vi "Inspect BBM Fiducials.vi"(5 "Dispose Images?":bool, 6 "BBM Chuck":i32, 7 "Glue Pathways":T7 {"BBM Slot" items=["Slot 1", "Slot 2", "Slot 3", "Slot 4"]; "Weight Slot" items=["Slot 1", "Slot 2", "Slot 3", "Slot 4"]; "Glue Slot" items=["Slot 1", "Slot 2", "Slot 3", "Slot 4"]; "Stamp Slot" items=["Slot 1", "Slot 2", "Slot 3", "Slot 4"]; "HDI Slot" items=["Slot 1", "Slot 2", "Slot 3", "Slot 4"]}, 8 "error in":errorcluster, 9 "Console Log in":refnum<class "Console Log.lvclass">, 10 "Single Path in":T6, 11 "CameraTool in":refnum<class "CameraTool Class.lvclass">) -> (0 "error out":errorcluster, 1 "Console Log out":refnum<class "Console Log.lvclass">, 2 "Single Path out":T6, 3 "CameraTool out":refnum<class "CameraTool Class.lvclass">)   [LabVIEW 2011, in "Gluing Procedure.lvclass"]
uses:
  Gluing Procedure.lvclass
  UI typedefs/Glue Path.ctl
  Shared Components/CameraTool Class/CameraTool Class.lvclass
  Shared Components/Utils/Type Definitions/Part Fiducials.ctl
  Shared Components/Utils/Type Definitions/Fiducial Image.ctl
  Shared Components/Vec3d Class/Vec3d Class.lvclass
  Shared Components/Utils/Type Definitions/Physical Image.ctl
  <vilib>/vision/Image Controls.llb/IMAQ Image.ctl
  Shared Components/Utils/Type Definitions/Fiducial with Source.ctl
  Application Utilities/Console Log/Console Log.lvclass
  Shared Components/Config Manager Class/Type Definitions/Part Type.ctl
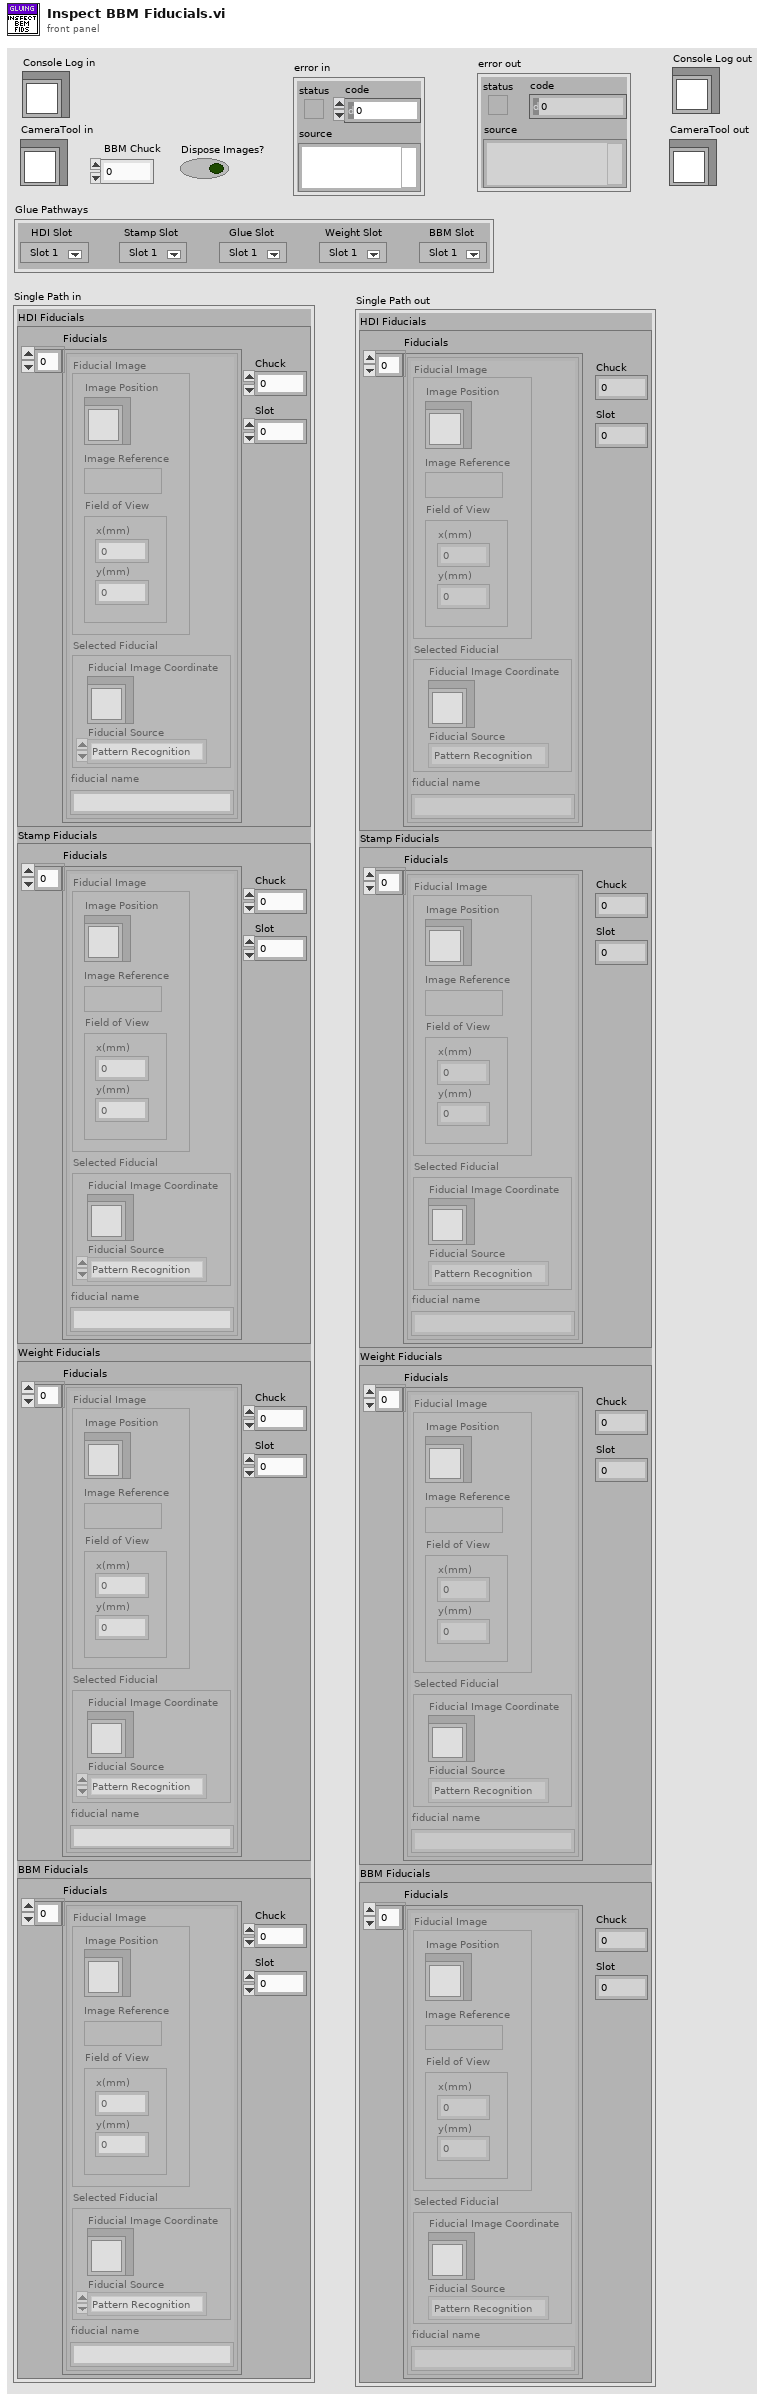
[diagram p1: front panel]
types:
  T1 = typedef "Part Fiducials.ctl" = cluster{"Fiducials":T2[], "Chuck":i32, "Slot":i32}
  T2 = typedef "Fiducial Image.ctl" = cluster{"Fiducial Image":T3, "Selected Fiducial":T5, "fiducial name":string}
  T3 = typedef "Physical Image.ctl" = cluster{"Image Position":refnum<class "Vec3d Class.lvclass">, "Image Reference":T4, "Field of View":cluster{"x(mm)":dbl, "y(mm)":dbl}}
  T4 = typedef "IMAQ Image.ctl" = refnum<image>
  T5 = typedef "Fiducial with Source.ctl" = cluster{"Fiducial Image Coordinate":refnum<class "Vec3d Class.lvclass">, "Fiducial Source":enum16{"Pattern Recognition", "User", "Error", "Default"}}
  T6 = cluster{"HDI Fiducials":T1, "Stamp Fiducials":T1, "Weight Fiducials":T1, "BBM Fiducials":T1}
  T7 = typedef "Glue Path.ctl" = cluster{"HDI Slot ":i32, "Stamp Slot":i32, "Glue Slot":i32, "Weight Slot":i32, "BBM Slot":i32}
  T8 = typedef "Part Type.ctl" = enum16{"BBM", "HDI", "BARE HDI", "GLUERESERVOIR", "STAMP_1", "STAMP_2", "STAMP_3", "STAMP_4", "STAMP_5", "WEIGHT_1", "WEIGHT_2", "WEIGHT_3", "WEIGHT_4", "WEIGHT_5", "WEIGHT_6", "WEIGHT_7", "WEIGHT_8", "PICKER_TOOL", "GRABER_TOOL"}
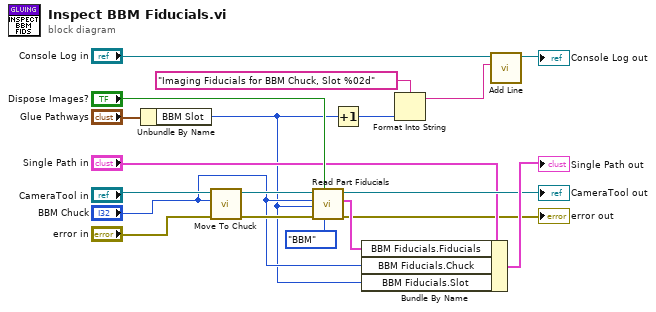
[diagram p0: block diagram]
diagram:
  n1 = Unbundle By Name("Glue Pathways") -> ("BBM Slot"=w1:i32)
  n2 = call-dynamic "Move To Chuck.vi"("error in"="error in", "Chuck"="BBM Chuck", "Gantry in"="CameraTool in") -> ("error out"=w10:errorcluster, "Gantry out"=w14:refnum<class "CameraTool Class.lvclass">)  [unwired: 7 in]
  n3 = call-dynamic "Read Part Fiducials.vi"("Part Type"=Part_Type."BBM", "Dispose Images?"="Dispose Images?", "error in"=w10, "Slot"=w1, "Chuck"="BBM Chuck", "CameraTool in"=w14) -> ("error out"=→"error out":errorcluster, "Fiducials"=w18:T2[], "CameraTool out"=→"CameraTool out":refnum<class "CameraTool Class.lvclass">)  [unwired: 3 in]
  n4 = Increment(x=w1) -> (x+1=w5:i32)
  n5 = Bundle By Name(cluster="Single Path in", "BBM Fiducials.Fiducials"=w18, "BBM Fiducials.Chuck"="BBM Chuck", "BBM Fiducials.Slot"=w1) -> (→"Single Path out":T6)
  n6 = Format Into String(format string="Imaging Fiducials for BBM Chuck, Slot %02d", w5) -> (resulting string=w3:string)  [unwired: 2 in, 1 out]
  n7 = call "Add Line.vi"("String"=w3, "Console Log in"="Console Log in") -> ("Console Log out"=→"Console Log out":refnum<class "Console Log.lvclass">)  [unwired: 8 in, 1 out]
